vi "Send RunningStatus Notifier.vi"(8 "error in (no error)":errorcluster, 10 "Running?":bool, 11 "Transport in":refnum<class "Transport.lvclass">) -> (0 "error out":errorcluster, 3 "Transport out":refnum<class "Transport.lvclass">)   [LabVIEW 2019, in "Transport.lvclass"]
uses:
  Transport.lvclass
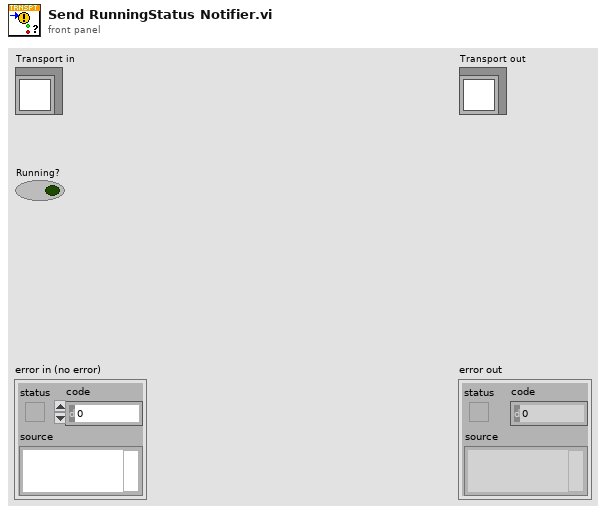
[diagram p1: front panel]
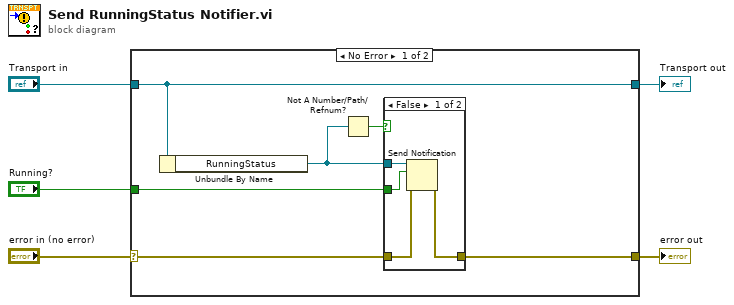
[diagram p0: block diagram]
diagram:
  n1 = case shown="No Error" "error in (no error)" {
    selector: "error in (no error)" -> [w11 w17]
    tunnel: [w10 w17] -> w4
    tunnel: [w9 w18] -> w2
    tunnel: "Transport in" -> [w9 w18]
    tunnel: "Running?" -> [w8 _]
    frame No Error {
      n2 = Unbundle By Name(w9) -> ("RunningStatus"=w7:refnum<notifier>)
      n3 = Not A Number/Path/Refnum?(number/path/refnum=w7) -> (NaN/Path/Refnum?=w6:bool)
      n4 = case shown="False" w6 {
        tunnel: w11 -> [w15 w16]
        tunnel: [w14 w16] -> w10
        tunnel: w8 -> [w13 _]
        tunnel: w7 -> [w12 _]
        frame False {
          n5 = Send Notification(notification=w13, notifier=w12, error in (no error)=w15) -> (error out=w14:errorcluster)  [unwired: 1 out]
        }
        frame True {
        }
      }
    }
    frame Error {
    }
  }
  "error out" <- w4
  "Transport out" <- w2
